vi "VotingRegressor.vi"(8 "error in":errorcluster) -> (0 "error out":errorcluster, 3 "out":refnum<class "VotingRegressor.lvclass">)   [LabVIEW 2020]
doc: "Prediction voting regressor for unfitted estimators.\n\n A voting regressor is an ensemble meta-estimator that fits several base\n regressors, each on the whole dataset. Then it averages the individual\n predictions to form a final prediction.\n\n Read more in the :ref:`User Guide <voting_regressor>`.\n\n .. versionadded:: 0.21\n\n Parameters\n ----------\n estimators : list of (str, estimator) tuples\n Invoking the ``fit`` method on the ``VotingRegressor`` will fit clones\n of those original estimators that will be stored in the class attribute\n ``self.estimators_``. An estimator can be set to ``'drop'`` using\n ``set_params``.\n\n .. versionchanged:: 0.21\n ``'drop'`` is accepted. Using None was deprecated in 0.22 and\n support was removed in 0.24.\n\n weights : array-like of shape (n_regressors,), default=None\n Sequence of weights (`float` or `int`) to weight the occurrences of\n predicted values before averaging. Uses uniform weights if `None`.\n\n n_jobs : int, default=None\n The number of jobs to run in parallel for ``fit``.\n ``None`` means 1 unless in a :obj:`joblib.parallel_backend` context.\n ``-1`` means using all processors. See :term:`Glossary <n_jobs>`\n for more details.\n\n verbose : bool, default=False\n If True, the time elapsed while fitting will be printed as it\n is completed.\n\n .. versionadded:: 0.23\n\n Attributes\n ----------\n estimators_ : list of regressors\n The collection of fitted sub-estimators as defined in ``estimators``\n that are not 'drop'.\n\n named_estimators_ : Bunch\n Attribute to access any fitted sub-estimators by name.\n\n .. versionadded:: 0.20\n\n See Also\n --------\n VotingClassifier : Soft Voting/Majority Rule classifier.\n\n \nAvailable methods:\nFit Transform\nTransform\nFit\nPredict\nScore\nGet Attributes\nGet Params\nSet Params"
uses:
  VotingRegressor.lvclass
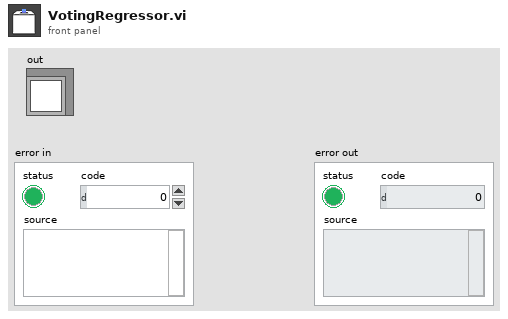
[diagram p1: front panel]
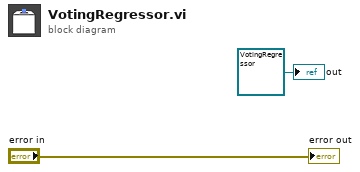
[diagram p0: block diagram]
diagram:
  "out" <- refnum<class "VotingRegressor.lvclass"> refnum ("model")
  "error out" <- "error in"
